vi "svl_Apply Highpass Filter with IC.vi"(6 "Initial Filter State":dbl[](array[numeric]) format="%.2f", 8 "error in (no error)":errorcluster, 9 "reset":bool, 10 "filter coefficients":T1 {"Forward Coefficients" format="%.4f"; "Reverse Coefficients" format="%.4f"}, 11 "signal [V]":dbl[](array[numeric])) -> (0 "error out":errorcluster, 3 "filtered signal [EU]":dbl[](array[numeric]), 4 "Final Filter State":dbl[](array[numeric]) format="%.2f")   [LabVIEW 2017, in "SoundVib_Integration.lvlib"]
uses:
  <vilib>/addons/Sound and Vibration/svt_Integration/SoundVib_Integration.lvlib
  <vilib>/Analysis/NI_AALBase.lvlib
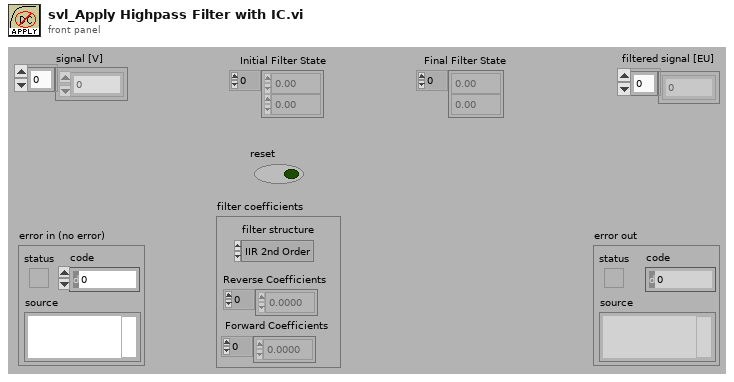
[diagram p1: front panel]
types:
  T1 = cluster{"filter structure":enum32{"IIR 2nd Order", "IIR 4th Order"}, "Reverse Coefficients":dbl[], "Forward Coefficients":dbl[]}
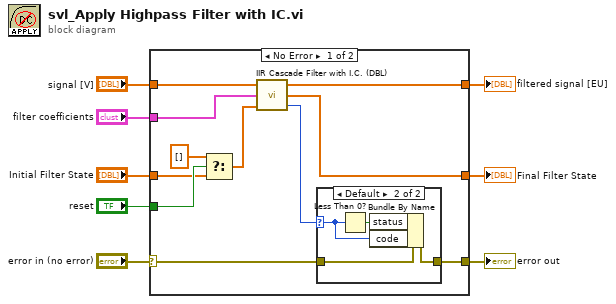
[diagram p0: block diagram]
diagram:
  n1 = case shown="No Error" "error in (no error)" {
    selector: "error in (no error)" -> [w19 w27]
    tunnel: "filter coefficients" -> [w15 _]
    tunnel: [w18 w27] -> w6
    tunnel: "reset" -> [w12 _]
    tunnel: "Initial Filter State" -> [w11 w26]
    tunnel: [w14 w26] -> w3
    tunnel: "signal [V]" -> [w17 w25]
    tunnel: [w16 w25] -> w1
    frame No Error {
      n2 = Select(t=dbl[] [], s=w12, f=w11) -> (s? t:f=w9:dbl[])
      n3 = call <vilib>:"IIR Cascade Filter with I.C. (DBL).vi"("Initial Filter State"=w9, "IIR Filter Cluster"=w15, "X"=w17) -> ("error"=w13:i32, "Final Filter State"=w14:dbl[], "Filtered X"=w16:dbl[])
      n4 = case shown="Default" w13 {
        selector: w13 -> [_ w21]
        tunnel: w19 -> [w20 w24]
        tunnel: [w20 w23] -> w18
        frame 0 {
        }
        frame Default {
          n5 = Less Than 0?(x=w21) -> (x < 0?=w22:bool)
          n6 = Bundle By Name(cluster=w24, "status"=w22, "code"=w21) -> (w23:errorcluster)
        }
      }
    }
    frame Error {
    }
  }
  "error out" <- w6
  "Final Filter State" <- w3
  "filtered signal [EU]" <- w1
